vi "AlliGator n-Exp + IRF Fit v4.vi"(0 "Decay":cluster{"t Array":dbl[], "Data Array":dbl[]}, 1 "VI Refnum":refnum<vi>, 2 "Optimal Offset Selection Criterion":T6, 5 "IRF":cluster{"t Array":dbl[], "IRF Array":dbl[]}, 7 "Fit Options":T17={"Show Fit Residuals"=TRUE, "Fit Model"=enum."1-Exponential", "Residual Type"=enum."Standard", "Max Decay Percentile"=0.0, "Min Decay Percentile"=0.0, "Show Full Decay"=TRUE, "Weights"=enum."Unweighted", "Fitting Method"=enum."Least Square", "Compute Parameter Uncertainties"=TRUE, "Periodic Boundaries"=TRUE, "Model Calculation"=enum."Simulation", "Period"=1.2500000000000001e-08, "Termination Criteria"={"Max Iterations"=1000, "Max Function Calls"=0, "Max Time"=1000.0, "Function Tolerance"=1e-06, "Parameter Tolerance"=1e-06, "Gradient Tolerance"=0.0, "Min Lambda"=1e-06, "Max Lambda"=1e-06, "Initial Tick Count"=0}, "Offset Resolution"=1.2500000000000001e-08, "Use Local IRF"=TRUE, "Fitting Algorithm"=enum."Levenberg-Marquardt", "Show Confidence Interval "=TRUE, "Confidence Level"=95.0} {"Confidence Level" min=0.0 max=100.0; "Offset Resolution" min=0.0; "Period" min=0.0; "Min Decay Percentile" min=0.0 max=1.0; "Max Decay Percentile" min=0.0 max=100.0}, 9 "MLE Fit Options":T7, 11 "error in (no error)":errorcluster, 12 "All Parameter Constraints":T16) -> (3 "All unscaled Fit Parameters (w tau)":dbl[](array[numeric]), 4 "Fit Plots":T5, 6 "Fit Control Data out":T1, 8 "Fit Output":T10={"best nonlinear fit"=[], "best fit parameters"=[], "R^2"=0.0, "RMSE"=0.0, "error out"={"status"=FALSE, "code"=0, "source"=""}, "Fitting Method"=enum."Least Square", "number of function calls"=0, "number of iterations"=0, "covariance"=[], "Chi 2"=0.0, "DOF"=0, "Fit Convergence Criterion"=enum."Continue", "Fitting Algorithm"=enum."Levenberg-Marquardt", "Weighted Fit"=enum."Unweighted", "Gradient"=0.0, "|Delta Chi 2|"=0.0, "|Delta Chi 2|/Chi 2"=0.0, "Max |Delta a| /|a|"=0.0, "Lambda"=-1.0, "RSS"=0.0, "AIC"=0.0, "BIC"=0.0, "Max number of function calls"=0, "Max number of iterations"=0, "IRF"={"X Array"=[], "Y Array"=[]}, "IRF Normalization Factor"=0.0, "Decay Normalization Factor"=0.0, "Number of offset fits"=0, "Weighted Chi2"=-1.0, "Unweighted Chi2"=-1.0}, 10 "Delta Best Fit Parameters (w tau)":dbl[](array[numeric]), 13 "Guess Parameters Options":T9=enum."User-provided (normalized)", 14 "Guess Parameters":dbl[](array[numeric]), 15 "error out":errorcluster)   [LabVIEW 2021, in "AlliGator Decay Fit.lvlib"]
doc: "Fits the provided decay to 1-Exp or 2-Exp model.\n\nThis VI assumes that <B>All Parameter Constraints</B> involve tau (rather than the square root of lifetime) and returns values with the same assumption."
uses:
  AlliGator Decay Fit.lvlib
  Time/Time.lvlib
  <vilib>/ErrorRing/Error Ring.xnode
  Fits/Fits.lvlib
  Globals, Variables, Constants/AlliGator Globals, Variables & Constants.lvlib
  Globals, Variables, Constants/AlliGator Variables List.ctl
  <vilib>/Utility/error.llb/Error Cluster From Error Code.vi
  Graphs/XY Graph/XY Graph Plot Data.ctl
  Graphs/XY Graph/XY Graph Add-Ons.lvlib
  Fits/IRF(X)PSED/Decay Fit Parameters In List.ctl
  Fits/Decay Convolution/Fit Control Data v2.ctl
  Fits/Decay Convolution/Decay Model.ctl
  Fits/Decay Fit Steps.ctl
  <vilib>/Analysis/Matrix/Datatypes/RealMatrix.ctl
  <vilib>/Analysis/Matrix/NI_Matrix.lvlib
  Fits/Convergence Criteria.ctl
  Fits/Non-linear Fitting Algorithm.ctl
  Fits/Non-linear Fit Output v4.ctl
  Fits/Fit Results (statistics).ctl
  Utilities/Utilities.lvlib
  Fits/Abort Fit Global.vi
  Fits/Non-linear Fitting Method v2.ctl
  Fits/Nonlinear Fit Method.ctl
  Error/Error.lvlib
  Fits/Fit Plots.ctl
  Fits/IRF(X)PSED/Fit Weights Type v2.ctl
  Fits/Residual Type.ctl
  Fits/Fit Calculation Method.ctl
  Fits/IRF(X)PSED/Decay Fit Parameter Constraints Arrays.ctl
  AlliGator Guess Parameters Options.ctl
  Fits/IRF(X)PSED/MLE Baseline Offset Type.ctl
  Fits/IRF(X)PSED/MLE Fit Options.ctl
  Fits/Optimal Offset Selection Criterion.ctl
  Fits/IRF(X)PSED/Decay Fit Options v4.ctl
panel:
  out "CPU (s)":dbl
  out "XY Graph":T21(graph)
  # "Offset\nBaseline\nAmplitude\nLifetime"
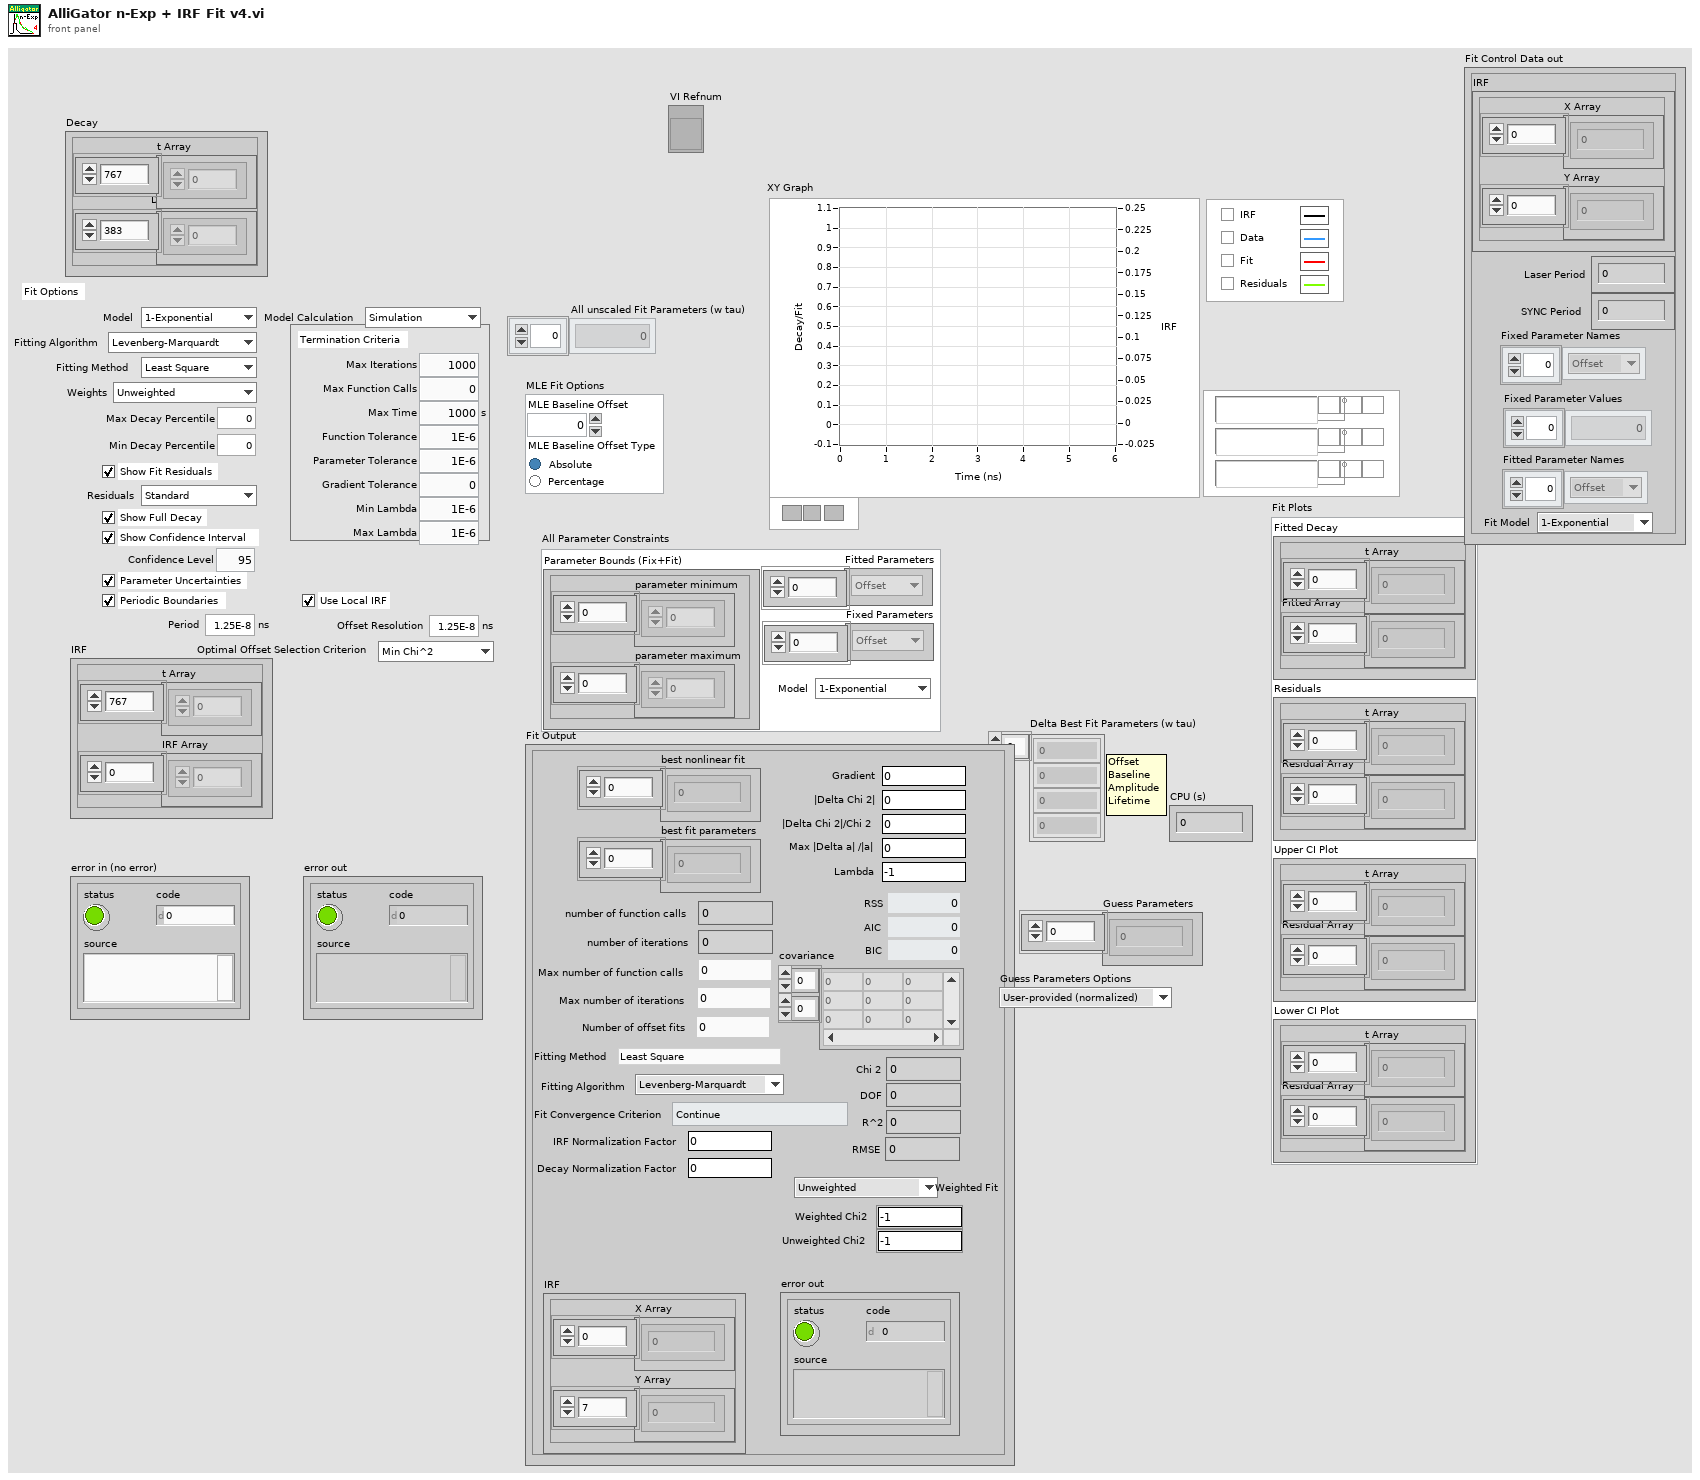
[diagram p1: front panel]
types:
  T1 = typedef "Fits.lvlib/Fit Control Data v2.ctl" = cluster{"IRF":T2, "Laser Period":dbl, "SYNC Period":dbl, "Fixed Parameter Names":T3[], "Fixed Parameter Values":dbl[], "Fitted Parameter Names":T3[], "Fit Model":T4}
  T2 = typedef "XY Graph Add-Ons.lvlib/XY Graph Plot Data.ctl" = cluster{"X Array":dbl[], "Y Array":dbl[]}
  T3 = typedef "Fits.lvlib/Decay Fit Parameters In List.ctl" = enum16{"Offset", "Baseline", "A_1", "tau_1", "A_2", "tau_2"}
  T4 = typedef "Fits.lvlib/Decay Model.ctl" = enum16{"1-Exponential", "2-Exponentials"}
  T5 = typedef "Fits.lvlib/Fit Plots.ctl" = cluster{"Fitted Decay":cluster{"t Array":dbl[], "Fitted Array":dbl[]}, "Residuals":cluster{"t Array":dbl[], "Residual Array":dbl[]}, "Upper CI Plot":cluster{"t Array":dbl[], "Residual Array":dbl[]}, "Lower CI Plot":cluster{"t Array":dbl[], "Residual Array":dbl[]}}
  T6 = typedef "Fits.lvlib/Optimal Offset Selection Criterion.ctl" = enum16{"Min Chi^2", "Max R^2"}
  T7 = typedef "Fits.lvlib/MLE Fit Options.ctl" = cluster{"MLE Baseline Offset":dbl, "MLE Baseline Offset Type":T8}
  T8 = typedef "Fits.lvlib/MLE Baseline Offset Type.ctl" = enum32{"Absolute", "Percentage"}
  T9 = typedef "AlliGator Decay Fit.lvlib/AlliGator Guess Parameters Options.ctl" = enum16{"Numerically estimated", "User-provided", "User-provided (normalized)", "Last valid fitted parameters"}
  T10 = typedef "Fits.lvlib/Non-linear Fit Output v4.ctl" = cluster{"best nonlinear fit":dbl[], "best fit parameters":dbl[], "R^2":dbl, "RMSE":dbl, "error out":errorcluster, "Fitting Method":T11, "number of function calls":i32, "number of iterations":i32, "covariance":T12, "Chi 2":dbl, "DOF":i32, "Fit Convergence Criterion":T13, "Fitting Algorithm":T14, "Weighted Fit":T15, "Gradient":dbl, "|Delta Chi 2|":dbl, "|Delta Chi 2|/Chi 2":dbl, "Max |Delta a| /|a|":dbl, "Lambda":dbl, "RSS":dbl, "AIC":dbl, "BIC":dbl, "Max number of function calls":i32, "Max number of iterations":i32, "IRF":T2, "IRF Normalization Factor":dbl, "Decay Normalization Factor":dbl, "Number of offset fits":i32, "Weighted Chi2":dbl, "Unweighted Chi2":dbl}
  T11 = typedef "Fits.lvlib/Nonlinear Fit Method.ctl" = enum16{"Least Square", "Least Absolute Residual", "Bisquare", "MLE"}
  T12 = typedef "NI_Matrix.lvlib/RealMatrix.ctl" = dbl[][]
  T13 = typedef "Fits.lvlib/Convergence Criteria.ctl" = enum16{"Continue", "Tolerances Exceeded", "Max Time Exceeded", "Max Iterations Exceeded", "Max Function Evaluations Exceeded", "Scale Range Exceeded"}
  T14 = typedef "Fits.lvlib/Non-linear Fitting Algorithm.ctl" = enum16{"Levenberg-Marquardt", "Trust-Region Dogleg"}
  T15 = typedef "Fits.lvlib/Fit Weights Type v2.ctl" = enum16{"Unweighted", "1/Variance (Neyman)", "1/Variance (Pearson)", "Best of All"}
  T16 = typedef "Fits.lvlib/Decay Fit Parameter Constraints Arrays.ctl" = cluster{"Parameter Bounds (Fix+Fit)":cluster{"parameter minimum":dbl[], "parameter maximum":dbl[]}, "Fitted Parameters":T3[], "Fixed Parameters":T3[], "Fit Model":T4}
  T17 = typedef "Fits.lvlib/Decay Fit Options v4.ctl" = cluster{"Show Fit Residuals":bool, "Fit Model":T4, "Residual Type":T18, "Max Decay Percentile":dbl, "Min Decay Percentile":dbl, "Show Full Decay":bool, "Weights":T15, "Fitting Method":T19, "Compute Parameter Uncertainties":bool, "Periodic Boundaries":bool, "Model Calculation":T20, "Period":dbl[unit], "Termination Criteria":cluster{"Max Iterations":i32, "Max Function Calls":i32, "Max Time":dbl[unit], "Function Tolerance":dbl, "Parameter Tolerance":dbl, "Gradient Tolerance":dbl, "Min Lambda":dbl, "Max Lambda":dbl, "Initial Tick Count":u32}, "Offset Resolution":dbl[unit], "Use Local IRF":bool, "Fitting Algorithm":T14, "Show Confidence Interval ":bool, "Confidence Level":dbl}
  T18 = typedef "Fits.lvlib/Residual Type.ctl" = enum16{"Standard", "Normalized", "Reduced"}
  T19 = typedef "Fits.lvlib/Non-linear Fitting Method v2.ctl" = enum16{"Least Square", "Least Absolute Residual", "Bisquare", "MLE", "-", "Best of All"}
  T20 = typedef "Fits.lvlib/Fit Calculation Method.ctl" = enum16{"Simulation", "Convolution", "Integration"}
  T21 = cluster{"t Array":dbl[], "best nonlinear fit":dbl[]}[]
  T22 = cluster{"parameter minimum":dbl[], "parameter maximum":dbl[]}
  T23 = cluster{"Max Iterations":i32, "Max Function Calls":i32, "Max Time":dbl[unit], "Function Tolerance":dbl, "Parameter Tolerance":dbl, "Gradient Tolerance":dbl, "Min Lambda":dbl, "Max Lambda":dbl, "Initial Tick Count":u32}
  T24 = typedef "Fits.lvlib/Decay Fit Steps.ctl" = enum16{"Unweighted Fit", "Weighted Fit", "Best Fit"}
  T25 = typedef "Fits.lvlib/Decay Fit Parameter Constraints with Values.ctl" = cluster{"Fitted parameter bounds":cluster{"parameter minimum":dbl[], "parameter maximum":dbl[]}, "Fixed Parameter Values":dbl[], "Fixed Parameter Names":T3[], "Fitted Parameter Names":T3[], "Fit Model":T4}
  T26 = typedef "Fits.lvlib/Fit Results (statistics).ctl" = cluster{"Chi2/DOF":dbl, "R2":dbl, "RMSE":dbl, "Fitting Method":T19, "Fitting Algorithm":T14}
  T27 = typedef "AlliGator Globals, Variables & Constants.lvlib/AlliGator Variables List.ctl" = enum16{"---- GUI ----", "GUI:Initialization Status", "GUI:State Indicators Refnum", "GUI:Original AlliGator Menu Items", "GUI:Current Action Loop State", "GUI:Script in progress", "GUI:Playback", "GUI:Loop Playback", "GUI:Search ROI Used", "GUI:Search ROI", "Decay Graph Max Legend Size", "Intensity Graph Max Legend Size", "Decay Statistics Graph Max Legend Size", "Phasor Graph Max Legend Size", "Phasor Ratio Graph Max Legend Size", "Lifetime Graph Max Legend Size", "---- Files ----", "Files:Export Dataset Frames as Individual Files", "Files:Show Batch Export Help Balloons", "Files:Frames in Dataset", "Files:ptu File Frame Start Indices", "Files:Current Frame in Dataset", "Files:Current Frame Timestamp", "Files:Dataset Loaded", "Files:Dataset Metadata", "Files:Dataset Channel", "Files:Dataset Data Description", "Files:Background Dataset Metadata", "Files:Background Dataset Channel", "Files:Background Dataset Data Description", "Files:Background File Subtraction", "Files:Background File Path", "Files:Background File Pile-up Correction", "Files:Background File Pixel Well Capacity", "Files:Background File Scaling Factor", "Files:Current Dataset Load Settings", "Files:Dataset Path", "Files:ICCD-specific Information", "Files:Macrotime Gate Separation", "------ Python Plugins ------", "Python Plugins:Information", "Python Plugins:Python Session", "Python Plugins:Valid Python Session?", "---- Source Image ----", "Source Image:ROIs", "Source Image:Current ROI", "Source Image:ROI Event Refnum", "X_Source Image:Display Range", "X_Source Image:Palette Information", "X_Source Image:Type of Displayed Image", "X_Time Gate Slider", "Source Image:Palette List", "Source Image:Scale", "Source Image:ROI Overlay Color", "Source Image:Overlay to Erase", "Source Image:Is Displayed Image Accumulated", "Source Image:White Light Image Modified", "Source Image:Mask Image Modified", "---- Image Profile Window ----", "Image Profile:Window Event Refnum", "Image Profile:IntensityType", "Image Profile:Intensity Average Type", "Image Profile:Intensity-weighted SDV", "Image Profile:Box Profile Type", "Image Profile:Window Open", "Image Profile:Plotted Fit Parameter", "------ Phasor Graph -------", "Phasor Graph:Show Line", "---- Phasor Plot ---", "Phasor Plot:Parameters Changed", "Phasor Plot:FLI Dataset Modified since last Calculation", "Phasor Harmonics Data", "Selected Phasor Harmonics", "Phasor Harmonic Manager Event Refnum", "Phasor Plot:ROIs", "Phasor Plot:Current ROI", "Phasor Plot:ROI Event Refnum", "Phasor Plot:Image Reference Points", "Phasor Plot:Computed", "Phasor Plot:Palette Information", "Phasor Plot:Palette List", "Phasor Plot:Phasor Ratio Palette Information", "Phasor Plot:Phasor Ratio Palette List", "Phasor Plot:Image Scale", "Phasor Plot:Image Overlay to Erase", "Phasor Plot:Image Elements to Update", "Phasor Plot:Current Calculation Parameters", "Phasor Plot:Current Calibration Options", "Phasor Plot:Reset Cumulated Phasor Plot", "Phasor Plot:Reference 1", "Phasor Plot:Lifetime Reference 1", "Phasor Plot:Reference 1 Frequency", "Phasor Plot:Reference 2", "Phasor Plot:Lifetime Reference 2", "Phasor Plot:Reference 2 Frequency", "---- Decay Analysis ----", "Number of Selected Decays to Fit", "LS Fit Results", "LAR Fit Results", "BS Fit Results", "Last Decay Max - Min", "Best Fit Parameters", "Best Fit Parameter Names", "Actual Size X", "Actual Size Y", "Binning X", "Binning Y", "Actual # Gates", "Dataset Number", "Gates to...", "Gates Skipped", "Gates to keep", "Gate Step", "Gate Separation", "Reversed Gates", "Pile-up Correction", "Pixel Well Capacity", "Background Subtracted", "Background Subtraction Method", "Background Definition Range", "Background File (deprecated)", "Number of Dataset Accumulated", "Array of Accumulated Dataset Paths", "Do Averaged Datasets", "Destination File Path", "Process Plot Target", "Use 1/D as Phasor Frequency", "---- Decay Fit Parameter Map -----", "Decay Fit Parameter Map:Palette Information", "Decay Fit Parameter Map:Palette List", "Decay Fit Parameter Map:X Resolution", "Decay Fit Parameter Map:Y Resolution", "Decay Fit Parameter Map:Use Decay Fit Result Constraints", "Decay Fit Parameter Map:Decay Fit Result Constraints", "Decay Fit Parameter Map:Decay Fit Result Constraints Applied", "---- Parameter Map ----", "Parameter Map:Palette Information", "Parameter Map:Palette List", "------- Local Decay Window ---------", "Local Decay Graph Window:Event Refnum", "Local Decay Graph Window:Use normalized IRF for convolution", "----- Miscellaneous ----", "Misc:Skippable Dialog Windows Status"}
  T28 = cluster{"t Array":dbl[], "best nonlinear fit":dbl[]}
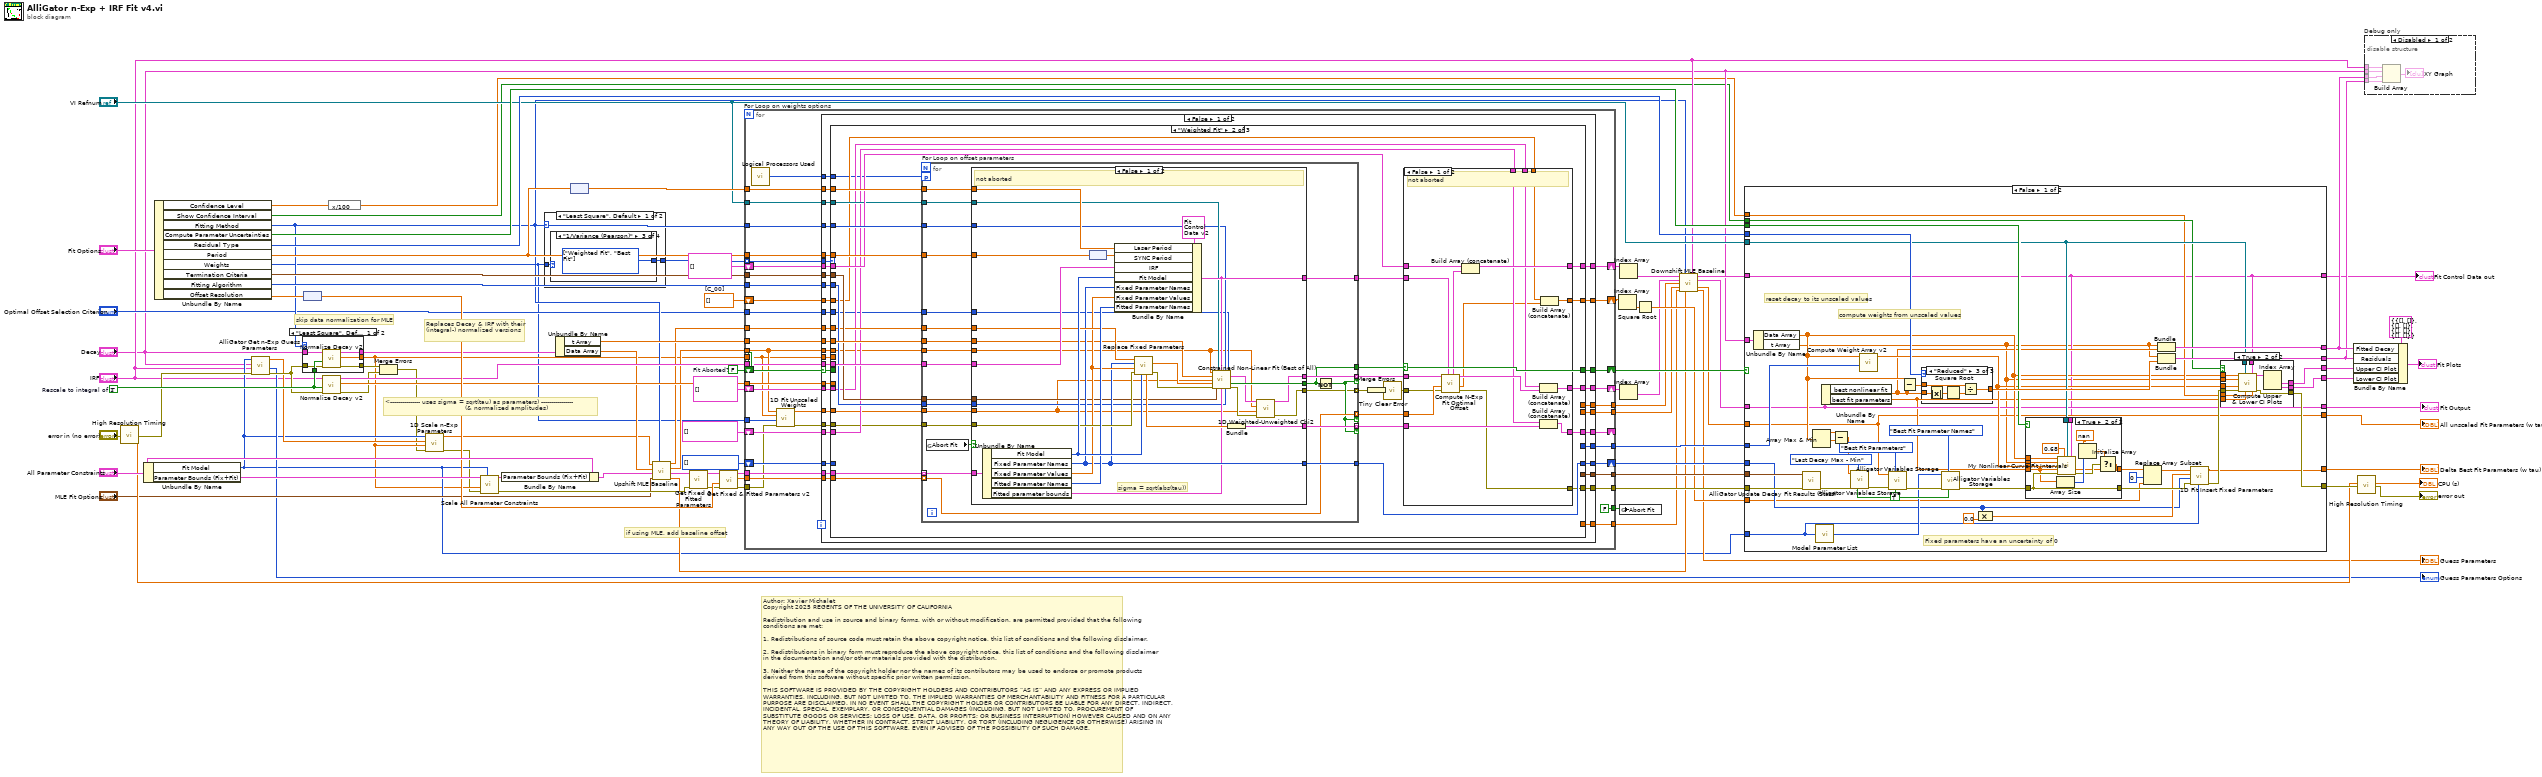
[diagram p0: block diagram]
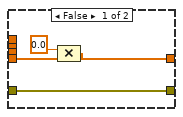
[diagram p4: hidden frame]
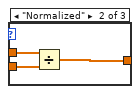
[diagram p6: hidden frame]
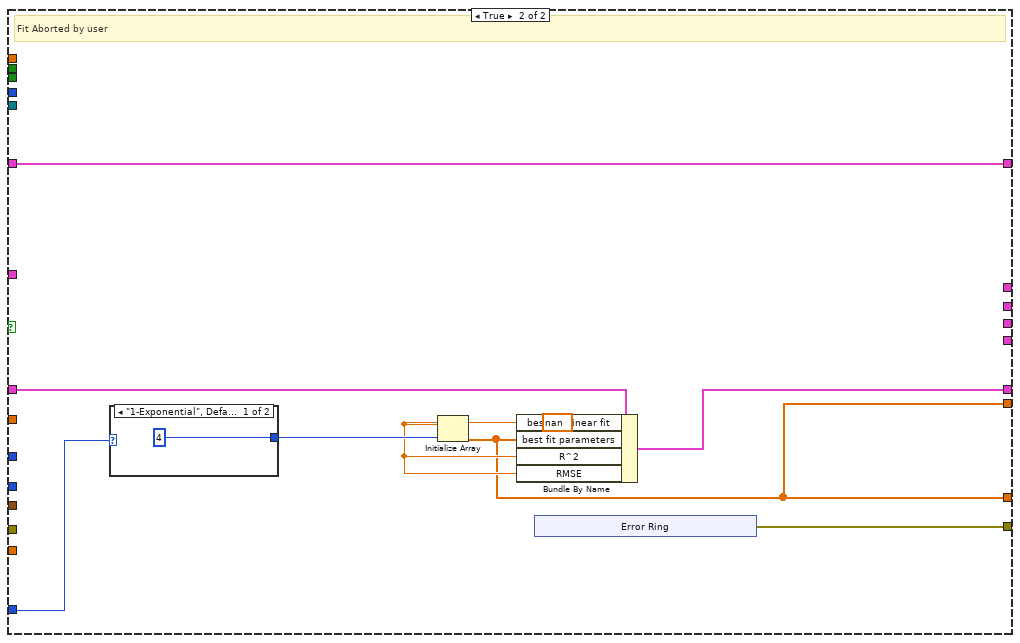
[diagram p7: hidden frame]
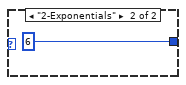
[diagram p8: hidden frame]
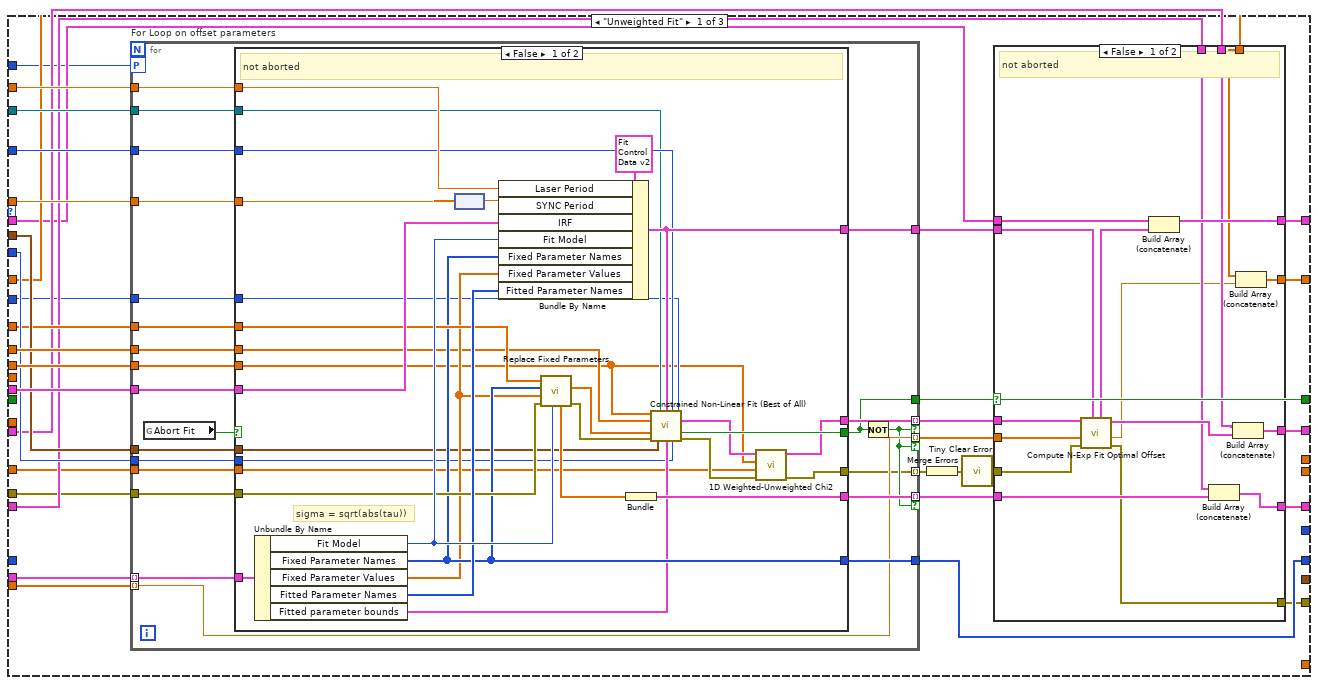
[diagram p9: hidden frame]
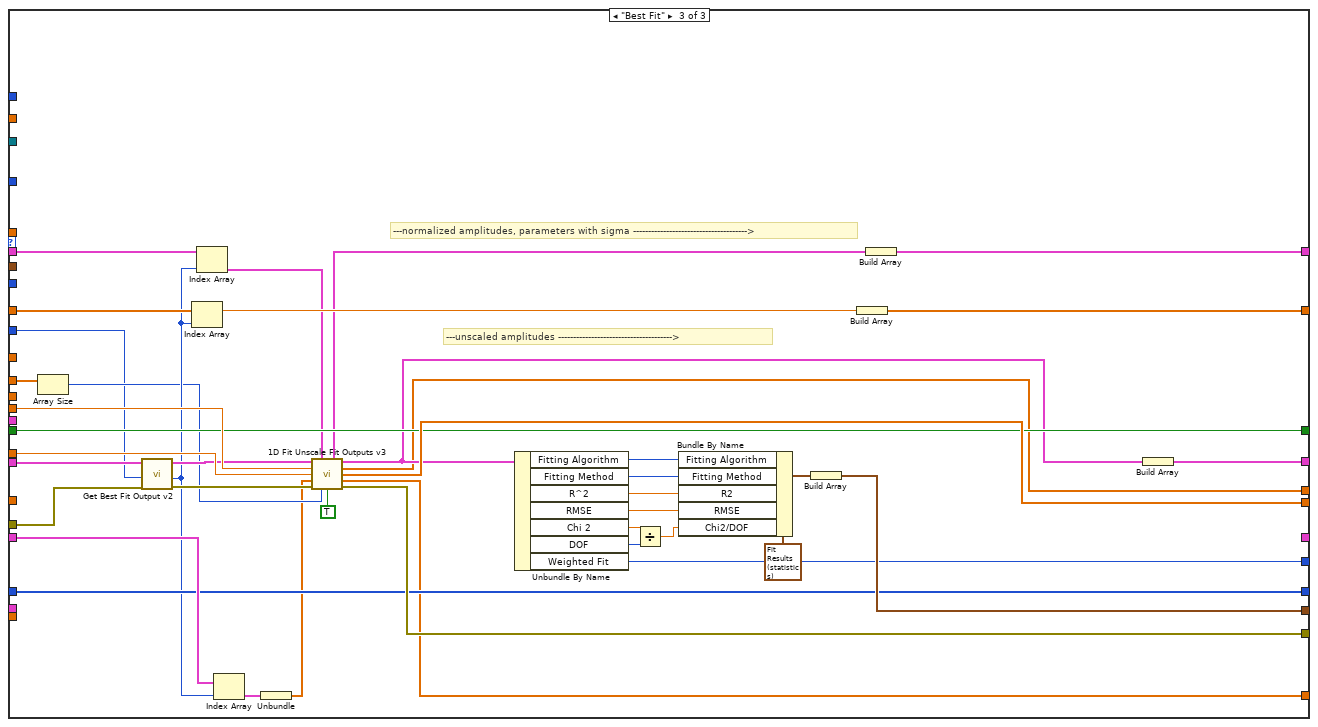
[diagram p14: hidden frame]
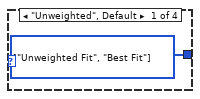
[diagram p16: hidden frame]
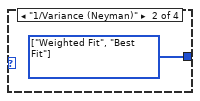
[diagram p17: hidden frame]
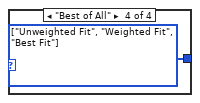
[diagram p18: hidden frame]
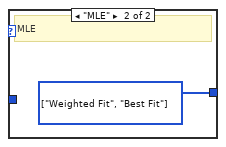
[diagram p19: hidden frame]
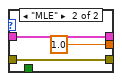
[diagram p20: hidden frame]
diagram:
  w54 = dbl[] []  # [C_00]
  w56 = T3[] [] items=["Offset", "Baseline", "A_1", "tau_1", "A_2", "tau_2"] ("Fixed Parameter Names")
  w68 = FALSE  # Fit Aborted?
  w45 = TRUE  # Rescale to integral of 1
  # "Author: Xavier Michalet\nCopyright 2025 REGENTS OF THE UNIVERSITY OF CALIFORNIA\n\nRedistribution and use in source and binary forms, with or without modification, are permitted provided that the following conditions are met:\n\n1. Redistributions of source code must retain the above copyright notice, this list of conditions and the following disclaimer.\n\n2. Redistributions in binary form must reproduce the above copyright notice, this list of conditions and the following disclaimer in the documentation and/or other materials provided with the distribution.\n\n3. Neither the name of the copyright holder nor the names of its contributors may be used to endorse or promote products derived from this software without specific prior written permission.\n\nTHIS SOFTWARE IS PROVIDED BY THE COPYRIGHT HOLDERS AND CONTRIBUTORS “AS IS” AND ANY EXPRESS OR IMPLIED WARRANTIES, INCLUDING, BUT NOT LIMITED TO, THE IMPLIED WARRANTIES OF MERCHANTABILITY AND FITNESS FOR A PARTICULAR PURPOSE ARE DISCLAIMED. IN NO EVENT SHALL THE COPYRIGHT HOLDER OR CONTRIBUTORS BE LIABLE FOR ANY DIRECT, INDIRECT, INCIDENTAL, SPECIAL, EXEMPLARY, OR CONSEQUENTIAL DAMAGES (INCLUDING, BUT NOT LIMITED TO, PROCUREMENT OF SUBSTITUTE GOODS OR SERVICES; LOSS OF USE, DATA, OR PROFITS; OR BUSINESS INTERRUPTION) HOWEVER CAUSED AND ON ANY THEORY OF LIABILITY, WHETHER IN CONTRACT, STRICT LIABILITY, OR TORT (INCLUDING NEGLIGENCE OR OTHERWISE) ARISING IN ANY WAY OUT OF THE USE OF THIS SOFTWARE, EVEN IF ADVISED OF THE POSSIBILITY OF SUCH DAMAGE."
  # "if using MLE, add baseline offset"
  # "skip data normalization for MLE"
  # "Replaces Decay & IRF with their (integral-) normalized versions"
  # "<--------------- uses sigma = sqrt(tau) as parameters) ----------------\n                                        (& normalized amplitudes)"
  n1 = call "High Resolution Timing.vi"("Error In"="error in (no error)") -> ("elapsed (relative) seconds"=w75:dbl, "Error Out"=w22:errorcluster)  [unwired: 16 in, 1 out]
  n2 = Unbundle By Name("All Parameter Constraints") -> ("Fit Model"=w17:T4, "Parameter Bounds (Fix+Fit)"=w84:T22)
  n3 = Unbundle By Name("Fit Options") -> ("Confidence Level"=w4:dbl, "Show Confidence Interval"=w7:bool, "Fitting Method"=w27:T19, "Compute Parameter Uncertainties"=w71:bool, "Residual Type"=w70:T18, "Period"=w44:dbl[unit], "Weights"=w1:T15, "Termination Criteria"=w74:T23, "Fitting Algorithm"=w73:T14, "Offset Resolution"=w66:dbl[unit])
  n4 = call "AlliGator Get n-Exp Guess Parameters.vi"("Error In"=w22, "IRF"="IRF", "Decay"="Decay", "Fit Model"=w17) -> ("Error Out"=w21:errorcluster, "Guess Parameters Options"=→"Guess Parameters Options":T9, "Guess Parameters"=w19:dbl[])  [unwired: 5 in]
  n5 = case shown="\"Least Square\", Default" w27 {
    tunnel: "Decay" -> [w98 w101]
    tunnel: [w97 w101] -> w59
    tunnel: [w96 1.0 ("Normalization Factor")] -> w16
    tunnel: w45 -> [w95 _]
    tunnel: w21 -> [w94 w99]
    tunnel: [w93 w99] -> w41
    frame "Least Square", Default {
      n6 = call "Normalize Decay v2.vi"("Error In"=w94, "Max = 1 (F)/Integral = 1 (T)"=w95, "Decay"=w98) -> ("Error Out"=w93:errorcluster, "Normalization Factor"=w96:dbl, "Normalized Decay"=w97:cluster{"t Array":dbl[], "Y Array":dbl[]})  [unwired: 4 in, 2 out]
    }
    frame "MLE" {
    }
  }
  n7 = node(w66) -> (w65:dbl)
  n8 = call "Normalize Decay v2.vi"("Error In"=w21, "Max = 1 (F)/Integral = 1 (T)"=w45, "Decay"="IRF") -> ("Error Out"=w42:errorcluster, "Normalization Factor"=w46:dbl, "Normalized Decay"=w60:cluster{"t Array":dbl[], "Y Array":dbl[]})  [unwired: 4 in, 2 out]
  n9 = expression code="x/100"(w4) -> (w3:dbl)
  n10 = Merge Errors(w41, w42) -> (w15:errorcluster)
  n11 = call "1D Scale n-Exp Parameters.vi"("Error In"=w15, "||F||"=w16, "Guess Parameters in"=w19, "Fit Model"=w17) -> ("Error Out"=w14:errorcluster, "Guess Parameters out"=w18:dbl[])  [unwired: 6 in]
  n12 = call "Scale All Parameter Constraints.vi"("Fit Model"=w17, "Error In"=w14, "Normalization Factor"=w16, "parameter bounds in (w tau)"=w84) -> ("Error Out"=w79:errorcluster, "parameter bounds out (w sigma)"=w82:T22)  [unwired: 6 in]
  n13 = Bundle By Name(cluster="All Parameter Constraints", "Parameter Bounds (Fix+Fit)"=w82) -> (w31:T16)
  n14 = case shown="\"Least Square\", Default" w27 {
    tunnel: w1 -> [w103 _]
    tunnel: [w102 w108] -> w76
    frame "Least Square", Default {
      n15 = case shown="\"1/Variance (Pearson)\"" w103 {
        tunnel: [w104 w105 w106 w107] -> w102
        frame "Unweighted", Default {
          w104 = T24[] [enum."Unweighted Fit", enum."Best Fit"] items=["Unweighted Fit", "Weighted Fit", "Best Fit"]
        }
        frame "1/Variance (Neyman)" {
          w105 = T24[] [enum."Weighted Fit", enum."Best Fit"] items=["Unweighted Fit", "Weighted Fit", "Best Fit"]
        }
        frame "1/Variance (Pearson)" {
          w106 = T24[] [enum."Weighted Fit", enum."Best Fit"] items=["Unweighted Fit", "Weighted Fit", "Best Fit"]
        }
        frame "Best of All" {
          w107 = T24[] [enum."Unweighted Fit", enum."Weighted Fit", enum."Best Fit"] items=["Unweighted Fit", "Weighted Fit", "Best Fit"]
        }
      }
    }
    frame "MLE" {
      w108 = T24[] [enum."Weighted Fit", enum."Best Fit"] items=["Unweighted Fit", "Weighted Fit", "Best Fit"]
      # "MLE"
    }
  }
  n16 = Unbundle By Name(w59) -> ("t Array"=w87:dbl[], "Data Array"=w32:dbl[])
  n17 = node(w44) -> (w88:dbl)
  n18 = call "Upshift MLE Baseline.vi"("NL Fit Method"=w27, "MLE Fit Options"="MLE Fit Options", "All Parameter Constraints in"=w31, "Data in"=w32, "Guess parameters in"=w18) -> ("MLE_Baseline_Offset out"=w26:dbl, "All Parameter Constraints out"=w28:T16, "Data out"=w29:dbl[], "Guess parameters out"=w30:dbl[])  [unwired: 3 in]
  n19 = call "Get Fixed & Fitted Parameters.vi"("Error In"=w79, "All Parameter Constraints"=w28) -> ("Error Out"=w62:errorcluster, "All Parameter Constraints with Values"=w78:T25)  [unwired: 8 in]
  n20 = call "Get Fixed & Fitted Parameters v2.vi"("Error In"=w62, "Offset Resolution"=w65, "All Parameter Constraints with Values"=w78) -> ("Error Out"=w61:errorcluster, "Offset Array"=w57:dbl[], "Array of Fit Parameter Constraints with Values"=w77:T25[])  [unwired: 5 in, 1 out]
  n21 = for "For Loop on weights options" {
    tunnel: w88 -> [w148]
    tunnel: w87 -> [w147]
    tunnel: w29 -> [w114]
    tunnel: w60 -> [w145]
    tunnel: w44 -> [w144]
    tunnel: [w143] -> w36
    tunnel: [w142] -> w34
    tunnel: [w141] -> w80
    tunnel: w46 -> [w140]
    tunnel: w16 -> [w113]
    tunnel: w77 -> [w139]
    tunnel: w76 -> [w138] mode=indexing
    tunnel: [w146] -> w58
    tunnel: w27 -> [w137]
    tunnel: w74 -> [w136]
    tunnel: w73 -> [w135]
    shift-right: [w134] -> w51
    shift-left: T10[] [] -> [w133]
    shift-right: [w132] -> w53
    shift-left: T1[] [] -> [w131]
    tunnel: "VI Refnum" -> [w130]
    tunnel: w30 -> [w129]
    shift-right: [w128] -> _
    shift-left: cluster{"All Guess Parameters (w tau)":dbl[]}[] [] -> [w127]
    shift-right: [w126] -> w55
    shift-left: w56 -> [w125]
    shift-right: [w124] -> w67
    shift-left: w68 -> [w123]
    tunnel: [w122] -> w64
    tunnel: w61 -> [w112]
    tunnel: w57 -> [w121]
    shift-right: [w120] -> w52
    shift-left: w54 -> [w119]
    tunnel: [FALSE ("Abort Fit")] -> w48
    tunnel: [w116] -> w24
    tunnel: "Optimal Offset Selection Criterion" -> [w115]
    tunnel: w1 -> [w109]
    n22 = call "Logical Processors Used.vi"() -> ("# Logical Processor Used"=w117:i32)  [unwired: 6 in]
    n23 = call "1D Fit Unscaled Weights.vi"("error in (no error)"=w112, "Weighted Fit"=w109, "Normalization Factor"=w113, "Data Array"=w114) -> ("error out"=w111:errorcluster, "Scaled Weight Array"=w110:dbl[])  [unwired: 6 in]
    n24 = case shown="False" w123 {
      selector: w123 -> [w158 w450]
      tunnel: w148 -> [w185 _]
      tunnel: w147 -> [w184 _]
      tunnel: w114 -> [w183 _]
      tunnel: [w182 _] -> w146
      tunnel: w145 -> [w181 _]
      tunnel: w144 -> [w180 _]
      tunnel: [w179 _] -> w143
      tunnel: [w178 _] -> w142
      tunnel: [w177 _] -> w141
      tunnel: w140 -> [w176 _]
      tunnel: w113 -> [w175 _]
      tunnel: w139 -> [w174 _]
      tunnel: w138 -> [w173 _]
      tunnel: w137 -> [w172 _]
      tunnel: w136 -> [w171 _]
      tunnel: w135 -> [w170 _]
      tunnel: [w169 _] -> w134
      tunnel: w133 -> [w168 _]
      tunnel: [w167 _] -> w132
      tunnel: w131 -> [w166 _]
      tunnel: w130 -> [w165 _]
      tunnel: w129 -> [w164 _]
      tunnel: [w163 _] -> w128
      tunnel: w127 -> [w162 _]
      tunnel: [w161 _] -> w126
      tunnel: w125 -> [w160 _]
      tunnel: [w159 w450] -> w124
      tunnel: [w157 _] -> w122
      tunnel: w121 -> [w156 _]
      tunnel: [w155 _] -> w120
      tunnel: w119 -> [w154 _]
      tunnel: w117 -> [w153 _]
      tunnel: [w152 _] -> w116
      tunnel: w115 -> [w151 _]
      tunnel: w111 -> [w150 _]
      tunnel: w110 -> [w149 _]
      frame False {
        n25 = case shown="\"Weighted Fit\"" w173 {
          tunnel: w185 -> [w219 w331 _]
          tunnel: w184 -> [w218 w330 w416]
          tunnel: w183 -> [w217 w307 _]
          tunnel: [w191 w302 w446] -> w182
          tunnel: w181 -> [w216 w329 _]
          tunnel: w180 -> [w215 w328 _]
          tunnel: [_ _ w444] -> w179
          tunnel: [_ _ w411] -> w178
          tunnel: [_ _ w445] -> w177
          tunnel: w176 -> [_ _ w447]
          tunnel: w175 -> [_ _ w448]
          tunnel: w174 -> [w214 w327 _]
          tunnel: w172 -> [w213 w326 _]
          tunnel: w171 -> [w212 w325 _]
          tunnel: w170 -> [w211 w324 _]
          tunnel: [w210 w306 w420] -> w169
          tunnel: w168 -> [w199 w312 w449]
          tunnel: [w209 w322 w424] -> w167
          tunnel: w166 -> [w190 w323 w443]
          tunnel: w165 -> [w208 w321 _]
          tunnel: w164 -> [w207 w320 _]
          tunnel: [w205 w318 _] -> w163
          tunnel: w162 -> [w198 w311 w442]
          tunnel: [w201 w314 w427] -> w161
          tunnel: w160 -> [_ _ w427]
          tunnel: [w197 w310 w441] -> w159
          tunnel: w158 -> [_ _ w441]
          tunnel: [_ _ w428] -> w157
          tunnel: w156 -> [w203 w316 _]
          tunnel: [w196 w308 w422] -> w155
          tunnel: w154 -> [w195 w309 w426]
          tunnel: w153 -> [w189 w298 _]
          tunnel: [_ _ w417] -> w152
          tunnel: w151 -> [w188 w301 w414]
          tunnel: w150 -> [w187 w300 w413]
          tunnel: w149 -> [w186 w299 _]
          frame "Unweighted Fit" {
            n26 = for "For Loop on offset parameters" {
              tunnel: w219 -> [w264]
              tunnel: [w252] -> w200
              tunnel: w218 -> [w250]
              tunnel: w217 -> [w251]
              tunnel: w216 -> [w263]
              tunnel: w215 -> [w262]
              tunnel: w214 -> [w261] mode=indexing
              tunnel: w187 -> [w260]
              tunnel: w213 -> [w246]
              tunnel: w212 -> [w249]
              tunnel: w211 -> [w248]
              tunnel: [w259] -> w204 mode=indexing if=w253
              tunnel: w208 -> [w247]
              tunnel: w207 -> [w258]
              tunnel: [w257] -> w201
              tunnel: [w256] -> w206 mode=indexing if=w253
              tunnel: [w255] -> w197
              tunnel: [w254] -> w202 mode=indexing if=w253
              tunnel: w203 -> [w254] mode=indexing
              tunnel: [w244] -> w194 mode=indexing
              workers-P: w189 -> [_]
              tunnel: w188 -> [w243]
              tunnel: w186 -> [w242]
              n27 = global read "Abort Fit Global.vi" "Abort Fit"() -> (w245:bool)
              n28 = case shown="False" w245 {
                selector: w245 -> [_ w297]
                tunnel: w264 -> [w295 _]
                tunnel: w263 -> [w293 _]
                tunnel: w262 -> [w292 _]
                tunnel: w261 -> [w289 _]
                tunnel: w260 -> [w288 w296]
                tunnel: [w268 _] -> w259
                tunnel: w258 -> [w285 _]
                tunnel: [w284 _] -> w257
                tunnel: [w282 _] -> w256
                tunnel: [w281 w297] -> w255
                tunnel: [w280 _] -> w252
                tunnel: w251 -> [w266 _]
                tunnel: w250 -> [w276 _]
                tunnel: w249 -> [w275 _]
                tunnel: w248 -> [w274 _]
                tunnel: w247 -> [w272 _]
                tunnel: w246 -> [w273 _]
                tunnel: [w267 w296] -> w244
                tunnel: w243 -> [w269 _]
                tunnel: w242 -> [w265 _]
                frame False {
                  # "sigma = sqrt(abs(tau))"
                  # "not aborted"
                  n29 = Unbundle By Name(w289) -> ("Fit Model"=w291:T4, "Fixed Parameter Names"=w284:T3[], "Fixed Parameter Values"=w277:dbl[], "Fitted Parameter Names"=w290:T3[], "Fitted parameter bounds"=w278:T22)
                  n30 = node(w292) -> (w294:dbl)
                  n31 = Bundle By Name(cluster=T1 {"IRF"={"X Array"=[], "Y Array"=[]}, "Laser Period"=0.0, "SYNC Period"=0.0, "Fixed Parameter Names"=[], "Fixed Parameter Values"=[], "Fitted Parameter Names"=[], "Fit Model"=enum."1-Exponential"}, "Laser Period"=w295, "SYNC Period"=w294, "IRF"=w293, "Fit Model"=w291, "Fixed Parameter Names"=w284, "Fixed Parameter Values"=w277, "Fitted Parameter Names"=w290) -> (w280:T1)
                  n32 = call "Replace Fixed Parameters.vi"("Fit Model"=w291, "Error In"=w288, "Fixed Parameter Values (w sigma)"=w277, "Fixed Parameter Names"=w284, "All Guess Parameters in (w tau)"=w285) -> ("Error Out"=w287:errorcluster, "Guess Fitted Parameters (w sigma)"=w279:dbl[], "All Guess Parameters (w tau)"=w283:dbl[])  [unwired: 2 in, 2 out]
                  n33 = Bundle("All Guess Parameters (w tau)"=w283) -> (w282:cluster{"All Guess Parameters (w tau)":dbl[]})  [unwired: 1 in]
                  n34 = call "Constrained Non-Linear Fit (Best of All).vi"("Y Array"=w266, "f(x,a)"=w272, "Data"=w280, "Fitting Method"=w273, "Optimal Offset Selection Criterion"=w269, "X Array"=w276, "Guess Fitted Parameters"=w279, "error in (no error)"=w287, "Termination Criteria"=w275, "Fitted parameter bounds"=w278, "Fitting Algorithm"=w274) -> ("Fit Output"=w270:T10, "Fit Aborted?"=w281:bool, "Error Out"=w271:errorcluster)  [unwired: 1 in, 1 out]
                  n35 = call "1D Weighted-Unweighted Chi2.vi"("error in (no error)"=w271, "Weight Array"=w265, "Y Array"=w266, "Fit Output"=w270) -> ("error out"=w267:errorcluster, "NL Fit Output"=w268:T10)  [unwired: 6 in]
                }
                frame True {
                  # "Fit aborted"
                }
              }
              n36 = Not(x=w255) -> (.not. x?=w253:bool)
            }
            n37 = Merge Errors(w194) -> (w193:errorcluster)
            n38 = call "Tiny Clear Error.vi"("Error In"=w193) -> ("no Error Out"=w192:errorcluster)  [unwired: 8 in]
            n39 = case shown="False" w197 {
              tunnel: [w236 w240] -> w210
              tunnel: w190 -> [w235 w241]
              tunnel: [w234 w241] -> w209
              tunnel: w206 -> [w233 _]
              tunnel: [w232 w239] -> w205
              tunnel: w204 -> [w231 _]
              tunnel: w202 -> [w230 _]
              tunnel: w200 -> [w222 _]
              tunnel: w199 -> [w228 w240]
              tunnel: w198 -> [w227 w239]
              tunnel: [w225 w238] -> w196
              tunnel: w195 -> [w224 w238]
              tunnel: w192 -> [w221 w237]
              tunnel: [w220 w237] -> w191
              frame False {
                # "not aborted"
                n40 = call "Compute N-Exp Fit Optimal Offset.vi"("Fit Control Data in"=w222, "Error In"=w221, "Offset Array"=w230, "Fit Output in"=w231) -> ("Error Out"=w220:errorcluster, "C_00"=w226:dbl, "Fit Output out"=w229:T10, "Fit Control Data out"=w223:T1)  [unwired: 4 in]
                n41 = Build Array (concatenate)(w235, w223) -> (w234:T1[])
                n42 = Build Array (concatenate)(w227, w233) -> (w232:cluster{"All Guess Parameters (w tau)":dbl[]}[])
                n43 = Build Array (concatenate)(w228, w229) -> (w236:T10[])
                n44 = Build Array (concatenate)(w224, w226) -> (w225:dbl[])
              }
              frame True {
                # "Fit aborted"
              }
            }
          }
          frame "Weighted Fit" {
            n45 = for "For Loop on offset parameters" {
              tunnel: w331 -> [w376]
              tunnel: [w364] -> w313
              tunnel: w330 -> [w362]
              tunnel: w307 -> [w363]
              tunnel: w329 -> [w375]
              tunnel: w328 -> [w374]
              tunnel: w327 -> [w373] mode=indexing
              tunnel: w300 -> [w372]
              tunnel: w326 -> [w358]
              tunnel: w325 -> [w361]
              tunnel: w324 -> [w360]
              tunnel: [w371] -> w317 mode=indexing if=w365
              tunnel: w321 -> [w359]
              tunnel: w320 -> [w370]
              tunnel: [w369] -> w314
              tunnel: [w368] -> w319 mode=indexing if=w365
              tunnel: [w367] -> w310
              tunnel: [w366] -> w315 mode=indexing if=w365
              tunnel: w316 -> [w366] mode=indexing
              tunnel: [w356] -> w305 mode=indexing
              tunnel: w301 -> [w355]
              tunnel: w299 -> [w354]
              workers-P: w298 -> [_]
              n46 = global read "Abort Fit Global.vi" "Abort Fit"() -> (w357:bool)
              n47 = case shown="False" w357 {
                selector: w357 -> [_ w409]
                tunnel: w376 -> [w407 _]
                tunnel: w375 -> [w405 _]
                tunnel: w374 -> [w404 _]
                tunnel: w373 -> [w401 _]
                tunnel: w372 -> [w400 w408]
                tunnel: [w381 _] -> w371
                tunnel: w370 -> [w397 _]
                tunnel: [w395 _] -> w369
                tunnel: [w393 _] -> w368
                tunnel: [w392 w409] -> w367
                tunnel: [w391 _] -> w364
                tunnel: w363 -> [w377 _]
                tunnel: w362 -> [w386 _]
                tunnel: w361 -> [w385 _]
                tunnel: w360 -> [w384 _]
                tunnel: w359 -> [w388 _]
                tunnel: w358 -> [w387 _]
                tunnel: [w379 w408] -> w356
                tunnel: w355 -> [w383 _]
                tunnel: w354 -> [w378 _]
                frame False {
                  # "sigma = sqrt(abs(tau))"
                  # "not aborted"
                  n48 = Unbundle By Name(w401) -> ("Fit Model"=w403:T4, "Fixed Parameter Names"=w395:T3[], "Fixed Parameter Values"=w396:dbl[], "Fitted Parameter Names"=w402:T3[], "Fitted parameter bounds"=w389:T22)
                  n49 = node(w404) -> (w406:dbl)
                  n50 = Bundle By Name(cluster=T1 {"IRF"={"X Array"=[], "Y Array"=[]}, "Laser Period"=0.0, "SYNC Period"=0.0, "Fixed Parameter Names"=[], "Fixed Parameter Values"=[], "Fitted Parameter Names"=[], "Fit Model"=enum."1-Exponential"}, "Laser Period"=w407, "SYNC Period"=w406, "IRF"=w405, "Fit Model"=w403, "Fixed Parameter Names"=w395, "Fixed Parameter Values"=w396, "Fitted Parameter Names"=w402) -> (w391:T1)
                  n51 = call "Replace Fixed Parameters.vi"("Fit Model"=w403, "Error In"=w400, "Fixed Parameter Values (w sigma)"=w396, "Fixed Parameter Names"=w395, "All Guess Parameters in (w tau)"=w397) -> ("Error Out"=w399:errorcluster, "Guess Fitted Parameters (w sigma)"=w390:dbl[], "All Guess Parameters (w tau)"=w394:dbl[])  [unwired: 2 in, 2 out]
                  n52 = call "Constrained Non-Linear Fit (Best of All).vi"("Y Array"=w377, "f(x,a)"=w388, "Data"=w391, "Fitting Method"=w387, "Optimal Offset Selection Criterion"=w383, "X Array"=w386, "Weights"=w378, "Guess Fitted Parameters"=w390, "error in (no error)"=w399, "Termination Criteria"=w385, "Fitted parameter bounds"=w389, "Fitting Algorithm"=w384) -> ("Fit Output"=w382:T10, "Fit Aborted?"=w392:bool, "Error Out"=w380:errorcluster)  [unwired: 1 out]
                  n53 = Bundle("All Guess Parameters (w tau)"=w394) -> (w393:cluster{"All Guess Parameters (w tau)":dbl[]})  [unwired: 1 in]
                  n54 = call "1D Weighted-Unweighted Chi2.vi"("error in (no error)"=w380, "Weight Array"=w378, "Y Array"=w377, "Fit Output"=w382) -> ("error out"=w379:errorcluster, "NL Fit Output"=w381:T10)  [unwired: 6 in]
                }
                frame True {
                  # "fit aborted"
                }
              }
              n55 = Not(x=w367) -> (.not. x?=w365:bool)
            }
            n56 = Merge Errors(w305) -> (w304:errorcluster)
            n57 = call "Tiny Clear Error.vi"("Error In"=w304) -> ("no Error Out"=w303:errorcluster)  [unwired: 8 in]
            n58 = case shown="False" w310 {
              tunnel: [w348 w352] -> w306
              tunnel: w323 -> [w347 w353]
              tunnel: [w346 w353] -> w322
              tunnel: w319 -> [w345 _]
              tunnel: [w344 w351] -> w318
              tunnel: w317 -> [w343 _]
              tunnel: w315 -> [w342 _]
              tunnel: w313 -> [w341 _]
              tunnel: w312 -> [w339 w352]
              tunnel: w311 -> [w338 w351]
              tunnel: w309 -> [w336 w350]
              tunnel: [w335 w350] -> w308
              tunnel: w303 -> [w333 w349]
              tunnel: [w332 w349] -> w302
              frame False {
                # "not aborted"
                n59 = call "Compute N-Exp Fit Optimal Offset.vi"("Fit Control Data in"=w341, "Error In"=w333, "Offset Array"=w342, "Fit Output in"=w343) -> ("Error Out"=w332:errorcluster, "C_00"=w337:dbl, "Fit Output out"=w340:T10, "Fit Control Data out"=w334:T1)  [unwired: 4 in]
                n60 = Build Array (concatenate)(w347, w334) -> (w346:T1[])
                n61 = Build Array (concatenate)(w339, w340) -> (w348:T10[])
                n62 = Build Array (concatenate)(w338, w345) -> (w344:cluster{"All Guess Parameters (w tau)":dbl[]}[])
                n63 = Build Array (concatenate)(w336, w337) -> (w335:dbl[])
              }
              frame True {
                # "fit aborted"
              }
            }
          }
          frame "Best Fit" {
            # "---normalized amplitudes, parameters with sigma -------------------------------------->"
            # "---unscaled amplitudes -------------------------------------->"
            n64 = Array Size(array=w416) -> (size(s)=w415:i32)
            n65 = call "Get Best Fit Output v2.vi"("error in"=w413, "Optimal Offset Selection Criterion"=w414, "Array of Fit Outputs"=w449) -> ("Error Out"=w430:errorcluster, "optimal index"=w425:i32, "Best Fit Output"=w440:T10)  [unwired: 6 in]
            n66 = Index Array(array=w426, index=w425) -> (element=w423:dbl)
            n67 = Index Array(array=w443, index=w425) -> (element=w419:T1)
            n68 = Index Array(array=w442, index=w425) -> (element=w429:cluster{"All Guess Parameters (w tau)":dbl[]})
            n69 = Unbundle(w429) -> ("All Guess Parameters (w tau)"=w412:dbl[])
            n70 = call "1D Fit Unscale Fit Outputs v3.vi"("Fit Output in  (w sigma)"=w440, "Fit Control Data in"=w419, "Decay Normalization Factor"=w448, "IRF Normalization Factor"=w447, "Scaled guess parameters (w tau)"=w412, "Error In"=w430, "# Points"=w415, "Order Lifetimes (F)"=TRUE) -> ("Fit Control Data out (w sigma)"=w418:T1, "Unscaled Fit Output out (w sigma)"=w421:T10, "Fitted unscaled parameters (w tau)"=w417:dbl[], "All unscaled parameters (w tau)"=w444:dbl[], "Unscaled guess parameters (w tau)"=w411:dbl[], "Error Out"=w446:errorcluster)  [unwired: 2 in]
            n71 = Unbundle By Name(w421) -> ("Fitting Algorithm"=w433:T14, "Fitting Method"=w437:T11, "R^2"=w436:dbl, "RMSE"=w435:dbl, "Chi 2"=w434:dbl, "DOF"=w432:i32, "Weighted Fit"=w428:T15)
            n72 = Divide(x=w434, y=w432) -> (x/y=w431:dbl)
            n73 = Bundle By Name(cluster=T26 {"Chi2/DOF"=0.0, "R2"=0.0, "RMSE"=0.0, "Fitting Method"=enum."Least Square", "Fitting Algorithm"=enum."Levenberg-Marquardt"} ("Fit Results (Stats)"), "Fitting Algorithm"=w433, "Fitting Method"=w437, "R2"=w436, "RMSE"=w435, "Chi2/DOF"=w431) -> (w438:T26)
            n74 = Build Array(w438) -> (w445:T26[])
            n75 = Build Array(w423) -> (w422:dbl[])
            n76 = Build Array(w418) -> (w424:T1[])
            n77 = Build Array(w421) -> (w420:T10[])
          }
        }
      }
      frame True {
      }
    }
  }
  n78 = Index Array(array=w52) -> (element=w50:dbl)  [unwired: 1 in]
  n79 = Index Array(array=w53) -> (element=w40:T1)  [unwired: 1 in]
  n80 = Index Array(array=w51) -> (element=w39:T10)  [unwired: 1 in]
  n81 = global write "Abort Fit Global.vi" "Abort Fit"(w48) -> ()
  n82 = Square Root(x=w50) -> (sqrt(x)=w49:dbl)
  n83 = call "Downshift MLE Baseline.vi"("Fit Control Data in"=w40, "NL Fit Method"=w27, "IRF"="IRF", "rescaled, w sigma"=w39, "Fitted unscaled parameters (w tau)"=w24, "All unscaled parameters (w tau)"=w36, "All Guess Parameters (w tau)"=w34, "MLE_Baseline_Shift"=w26) -> ("Fit Control Data out"=w38:T1, "Fit Output"=w37:T10, "All unscaled Parameters (w tau)"=w35:dbl[], "All Guess Parameters (w tau)"=→"Guess Parameters":dbl[])  [unwired: 3 in, 1 out]
  n84 = case shown="False" w67 {
    tunnel: [w470 _] -> w9
    tunnel: [w464 w544] -> w92
    tunnel: [w451 w539] -> w91
    tunnel: [w469 _] -> w8
    tunnel: "VI Refnum" -> [w468 _]
    tunnel: w37 -> [w458 w543]
    tunnel: [w458 w542] -> w89
    tunnel: w58 -> [w492 _]
    tunnel: w80 -> [w484 _]
    tunnel: w35 -> [w456 _]
    tunnel: w55 -> [w473 _]
    tunnel: w70 -> [w479 _]
    tunnel: w71 -> [w478 _]
    tunnel: "Decay" -> [w477 _]
    tunnel: w38 -> [w455 w538]
    tunnel: w17 -> [w475 w540]
    tunnel: w64 -> [w474 _]
    tunnel: w49 -> [w453 _]
    tunnel: [w456 w539] -> w47
    tunnel: w7 -> [w463 _]
    tunnel: w3 -> [w462 _]
    tunnel: [w467 _] -> w6
    tunnel: [w466 _] -> w5
    tunnel: [w455 w538] -> w2
    frame False {
      w489 = TRUE ("Get(F)/Set")
      # "compute weights from unscaled values"
      # "reset decay to its unscaled values"
      # "Fixed parameters have an uncertainty of 0"
      n85 = Unbundle By Name(w477) -> ("Data Array"=w461:dbl[], "t Array"=w454:dbl[])
      n86 = call "AlliGator Update Decay Fit Results (Stats).vi"("error in (no error)"=w492, "Fit Results"=w484) -> ("error out"=w491:errorcluster)  [unwired: 9 in]
      n87 = Array Max & Min(array=w461) -> (max value=w487:dbl, min value=w486:dbl)  [unwired: 2 out]
      n88 = call "Model Parameter List.vi"("Fit Model"=w475) -> ("Model Parameter List"=w476:T3[])
      n89 = Unbundle By Name(w458) -> ("best nonlinear fit"=w459:dbl[], "best fit parameters"=w457:dbl[])
      n90 = Subtract(x=w487, y=w486) -> (x-y=w485:dbl)
      n91 = call "Alligator Variables Storage.vi"("Get(F)/Set"=w489, "AlliGator Variable"=AlliGator_Variables_List."Last Decay Max - Min" ("Alligator Variable"), "Error In"=w491, "Data in"=w485) -> ("Error Out"=w490:errorcluster)  [unwired: 5 in, 2 out]
      n92 = call "Compute Weight Array v2.vi"("Weighted Fit"=w474, "Data Array"=w461) -> ("Weight Array"=w460:dbl[])  [unwired: 8 in, 1 out]
      n93 = call "Alligator Variables Storage.vi"("Get(F)/Set"=w489, "AlliGator Variable"=AlliGator_Variables_List."Best Fit Parameters" ("Alligator Variable"), "Error In"=w490, "Data in"=w456) -> ("Error Out"=w494:errorcluster)  [unwired: 5 in, 2 out]
      n94 = Subtract(x=w461, y=w459) -> (x-y=w497:dbl[])
      n95 = case shown="\"Reduced\"" w479 {
        tunnel: w497 -> [w529 w532 w537]
        tunnel: [w529 w530 w535] -> w496
        tunnel: w459 -> [_ w531 w536]
        frame "Standard", Default {
        }
        frame "Normalized" {
          n96 = Divide(x=w532, y=w531) -> (x/y=w530:dbl[])
        }
        frame "Reduced" {
          n97 = Absolute Value(x=w536) -> (abs(x)=w534:dbl[])
          n98 = Square Root(x=w534) -> (sqrt(x)=w533:dbl[])
          n99 = Divide(x=w537, y=w533) -> (x/y=w535:dbl[])
        }
      }
      n100 = call "Alligator Variables Storage.vi"("Get(F)/Set"=w489, "AlliGator Variable"=AlliGator_Variables_List."Best Fit Parameter Names" ("Alligator Variable"), "Error In"=w494, "Data in"=w476) -> ("Error Out"=w483:errorcluster)  [unwired: 5 in, 2 out]
      n101 = Compound Arithmetic op=MULTIPLY(w473, 0.0 ("value")) -> (w481:dbl[])
      n102 = case shown="True" w478 {
        tunnel: [w514 w517] -> w482
        tunnel: [w511 w518] -> w472
        tunnel: w454 -> [_ w527]
        tunnel: w468 -> [_ w526]
        tunnel: w460 -> [_ w525]
        tunnel: w455 -> [_ w524]
        tunnel: w483 -> [w514 w517]
        tunnel: w457 -> [w512 w516]
        tunnel: w461 -> [_ w515]
        frame False {
          n103 = Compound Arithmetic op=MULTIPLY(0.0, w512) -> (w511:dbl[])
        }
        frame True {
          n104 = Array Size(array=w516) -> (size(s)=w523:i32)
          n105 = call "My Nonlinear Curve Fit Intervals.vi"("Y"=w515, "confidence level"=0.68, "f(x,a)"=w526, "data"=w524, "X"=w527, "Weight"=w525, "best fit parameters"=w516, "error in (no error)"=w517) -> ("delta best fit parameters"=w519:dbl[], "error out"=w520:errorcluster)  [unwired: 6 in]
          n106 = Initialize Array(nan ("element"), w523) -> (w521:dbl[])
          n107 = Select(t=w521, s=w520, f=w519) -> (s? t:f=w518:dbl[])
        }
      }
      n108 = Replace Array Subset(array=w472, new element=w453, index=0) -> (w471:dbl[])
      n109 = Bundle("t Array"=w454, "best nonlinear fit"=w459) -> (w470:T28)  [unwired: 1 in]
      n110 = Bundle("t Array"=w454, w496) -> (w469:cluster{"t Array":dbl[], dbl[]})  [unwired: 1 in]
      n111 = call "1D Fit Insert Fixed Parameters.vi"("Fit Model"=w475, "Error In"=w482, "Fixed Parameter Names"=w473, "Fixed Parameter Values"=w481, "Fitted Parameters"=w471) -> ("Error Out"=w465:errorcluster, "All Parameters"=w451:dbl[])  [unwired: 5 in]
      n112 = case shown="True" w463 {
        tunnel: w468 -> [_ w510]
        tunnel: w455 -> [_ w509]
        tunnel: [_ w507] -> w467
        tunnel: [_ w506] -> w466
        tunnel: w465 -> [w498 w500]
        tunnel: [w498 w505] -> w464
        tunnel: w462 -> [_ w504]
        tunnel: w461 -> [_ w503]
        tunnel: w454 -> [_ w502]
        tunnel: w460 -> [_ w501]
        tunnel: w457 -> [_ w499]
        frame False {
        }
        frame True {
          n113 = call "Compute Upper & Lower CI Plots.vi"("Y Array"=w503, "VI in"=w510, "Additional LM Data"=w509, "X Array"=w502, "Weight Array"=w501, "error in (no error)"=w500, "best fit parameters"=w499, "confidence level (0.95)"=w504) -> ("CI Plots"=w508:T2[], "error out"=w505:errorcluster)  [unwired: 6 in]
          n114 = Index Array(array=w508) -> (element #1=w507:T2, element #2=w506:T2)  [unwired: 2 in]
        }
      }
    }
    frame True {
      w541 = nan ("element")
      # "Fit Aborted by user"
      n115 = case shown="\"1-Exponential\", Default" w540 {
        tunnel: [4 ("dimension size") 6 ("dimension size")] -> w545
        frame "1-Exponential", Default {
        }
        frame "2-Exponentials" {
        }
      }
      n116 = Initialize Array(w541, w545) -> (w539:dbl[])
      n117 = Bundle By Name(cluster=w543, "best nonlinear fit"=w539, "best fit parameters"=w539, "R^2"=w541, "RMSE"=w541) -> (w542:T10)
      n118 = xnode "Error Ring"() -> ("error out"=w544:errorcluster)
    }
  }
  "Delta Best Fit Parameters (w tau)" <- w91
  "Fit Output" <- w89
  "All unscaled Fit Parameters (w tau)" <- w47
  "Fit Control Data out" <- w2
  n119 = Bundle By Name(cluster=T5 {"Fitted Decay"={"t Array"=[], "Fitted Array"=[]}, "Residuals"={"t Array"=[], "Residual Array"=[]}, "Upper CI Plot"={"t Array"=[], "Residual Array"=[]}, "Lower CI Plot"={"t Array"=[], "Residual Array"=[]}} ("Fit Plots"), "Fitted Decay"=w9, "Residuals"=w8, "Upper CI Plot"=w6, "Lower CI Plot"=w5) -> (→"Fit Plots":T5)
  n120 = call "High Resolution Timing.vi"("relative seconds (NaN)"=w75, "Error In"=w92) -> ("elapsed (relative) seconds"=→"CPU (s)":dbl, "Error Out"=→"error out":errorcluster)  [unwired: 15 in, 1 out]
  n121 = disable-structure "Debug only" shown="Disabled" {
    disable-tunnel: "IRF" -> [w556 _]
    disable-tunnel: "Decay" -> [w555 _]
    disable-tunnel: w9 -> [w554 _]
    disable-tunnel: w8 -> [w553 _]
    frame Disabled {
      n122 = Build Array(w556, w555, w554, w553) -> (→"XY Graph":T21)
    }
    frame Enabled {
    }
  }
